vi "Grab with Software Trigger - LV2014.vi"() -> ()   [LabVIEW 2014]
doc: "The Grab VI acquires images continuously and displays the images in an image control using high-level acquisition VIs. A grab is appropriate for high-speed applications in which you need to process only one image at a time."
uses:
  <vilib>/vision/driver/NI_Vision_Acquisition_Software.lvlib
  <resource>/objmgr/imaqdx.rc
panel:
  in  "Timeout (ms)":u32=5000
  in  "Send Trigger":bool
  in  "Camera Name":refnum<k21> caption="IMAQdx Session"
  out "Buffer Number":u32
  out "Image":T1(plugin-control)
  out "Frame Rate":dbl(knob)=1.0526315789473684 scale=0.0..100.0
  in  "Stop":bool
  # "Overview: Demonstrates how to acquire images a Grab acquisition with software triggering.\nRequirements: Vision Acquisition Software\nInstructions: \n1. Select the Camera Name.\n2. Set Timeout (ms) to a value high enough to allow time to generate the trigger.\n3. Run the VI.\n4. Click Send Trigger to trigger the acquisition of a frame.\n5. After clicking Stop, VI will wait the timeout duration before stopping."
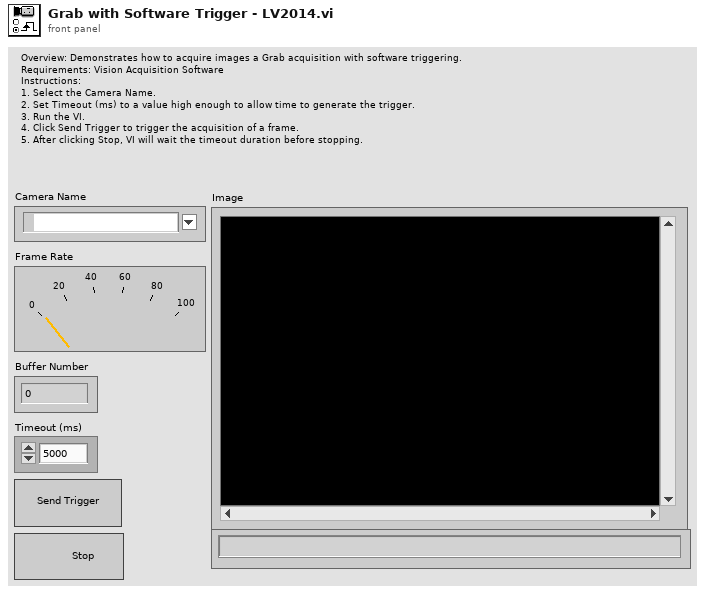
[diagram p1: front panel]
types:
  T1 = typedef "IMAQ Image.ctl" = refnum<image>
  T2 = typedef "IMAQdx.ctl" = refnum<k21>
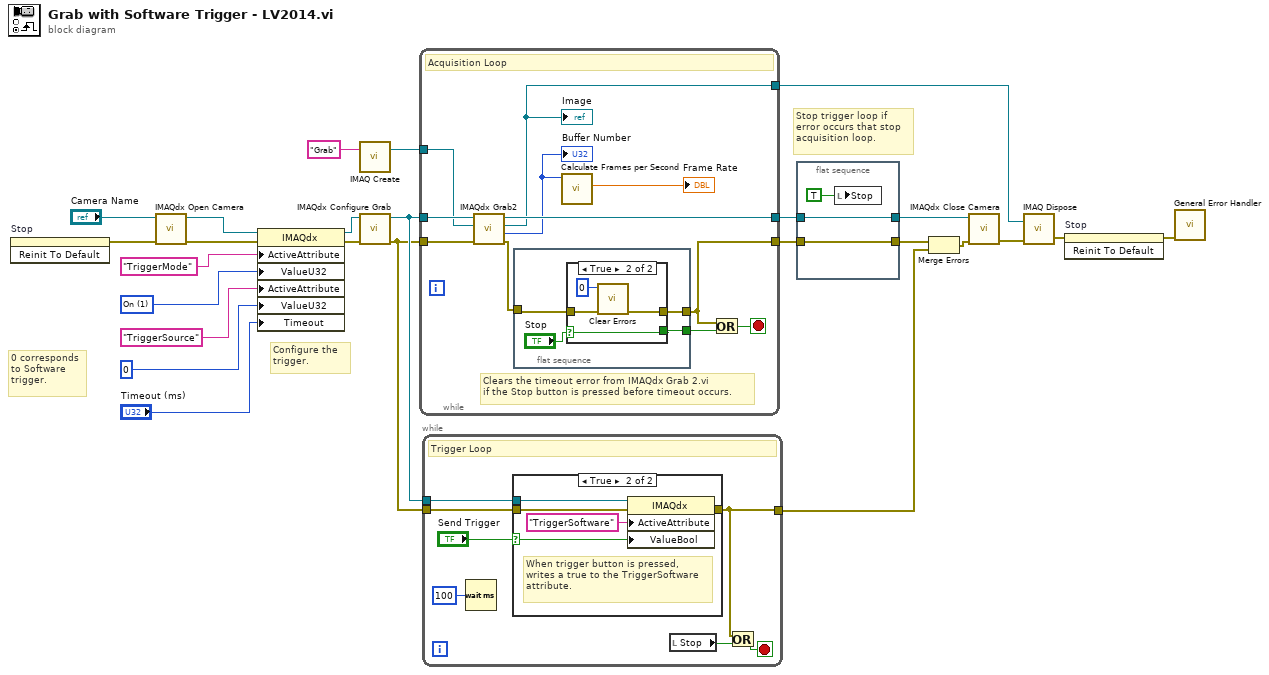
[diagram p0: block diagram]
diagram:
  w12 = u32 1 items=["Off", "On"] ("Trigger Mode")
  # "Configure the \ntrigger."
  # "Stop trigger loop if\nerror occurs that stop \nacquisition loop."
  # "0 corresponds\nto Software \ntrigger."
  n1 = invoke on="Stop" class="Bool (strict)" method="Reinit To Default"() -> (error out=w9:errorcluster)  [unwired: 3 in, 2 out]
  n2 = call <vilib>:"IMAQdx Open Camera.vi"("error in"=w9, "Session In"="Camera Name") -> ("error out"=w24:errorcluster, "Session Out"=w18:T2)  [unwired: 1 in, 7 out]
  n3 = property class="IMAQdx"(reference=w18, error in=w24, "ActiveAttribute"="TriggerMode", "ValueU32"=w12, "ActiveAttribute"="TriggerSource", "ValueU32"=u32 0, "Timeout"="Timeout (ms)") -> (reference out=w17:T2, error out=w19:errorcluster)
  n4 = call "IMAQ Create"("Image Name"="Grab") -> ("New Image"=w25:T1)  [unwired: 3 in, 2 out]
  n5 = call <vilib>:"IMAQdx Configure Grab.vi"("error in"=w19, "Session In"=w17) -> ("error out"=w10:errorcluster, "Session Out"=w11:T2)  [unwired: 8 out]
  n6 = while {
    tunnel: [w32] -> w8
    tunnel: w10 -> [w34]
    tunnel: w11 -> [w35]
    tunnel: [w26] -> w7
    tunnel: w25 -> [w33]
    tunnel: [w29] -> w22
    stop <- w36 stop-if-true
    # "Clears the timeout error from IMAQdx Grab 2.vi\nif the Stop button is pressed before timeout occurs."
    # "Acquisition Loop"
    n7 = call <vilib>:"IMAQdx Grab2.vi"("error in"=w34, "Image In"=w33, "Session In"=w35) -> ("error out"=w27:errorcluster, "Buffer Number Out"=w30:u32, "Image Out"=w29:T1, "Session Out"=w32:T2)  [unwired: 5 in]
    "Image" <- w29
    "Buffer Number" <- w30
    n8 = flat-sequence {
      tunnel: [w39] -> w28
      tunnel: w27 -> [w38]
      tunnel: [w37] -> w26
      frame #0 {
        n9 = case shown="True" "Stop" {
          selector: "Stop" -> [w41 w46]
          tunnel: [w41 w46] -> w39
          tunnel: w38 -> [w42 w45]
          tunnel: [w42 w44] -> w37
          frame False {
          }
          frame True {
            n10 = call <vilib>:"Clear Errors.vi"("error in (no error)"=w45, "specific error code to clear (0: all)"=0) -> ("error out"=w44:errorcluster)  [unwired: 4 in, 1 out]
          }
        }
      }
    }
    n11 = call <vilib>:"Calculate Frames per Second.vi"("Buffer Number"=w30) -> ("Processed Frames/s"=→"Frame Rate":dbl)  [unwired: 8 in, 2 out]
    n12 = Or(x=w26, y=w28) -> (x .or. y?=w36:bool)
  }
  n13 = while {
    tunnel: w11 -> [w52]
    tunnel: w10 -> [w51]
    tunnel: [w49] -> w1
    stop <- w50 stop-if-true
    # "Trigger Loop"
    n14 = Wait (ms)(milliseconds to wait=u32 100) -> ()  [unwired: 1 out]
    n15 = case shown="True" "Send Trigger" {
      selector: "Send Trigger" -> [_ w55]
      tunnel: w52 -> [_ w59]
      tunnel: w51 -> [w54 w58]
      tunnel: [w54 w57] -> w49
      frame False {
      }
      frame True {
        # "When trigger button is pressed,\nwrites a true to the TriggerSoftware\nattribute."
        n16 = property class="IMAQdx"(reference=w59, error in=w58, "ActiveAttribute"="TriggerSoftware", "ValueBool"=w55) -> (error out=w57:errorcluster)  [unwired: 1 out]
      }
    }
    n17 = local read "Stop"() -> (w53:bool)
    n18 = Or(x=w49, y=w53) -> (x .or. y?=w50:bool)
  }
  n19 = flat-sequence {
    tunnel: w8 -> [w60]
    tunnel: w7 -> [w61]
    tunnel: [w61] -> w6
    tunnel: [w60] -> w5
    frame #0 {
      n20 = local write "Stop"(TRUE ("Stop")) -> ()
    }
  }
  n21 = Merge Errors(w6, w1) -> (w2:errorcluster)
  n22 = call <vilib>:"IMAQdx Close Camera.vi"("error in"=w2, "Session In"=w5) -> ("error out"=w21:errorcluster)  [unwired: 9 out]
  n23 = call "IMAQ Dispose"("Image"=w22, "error in (no error)"=w21) -> ("error out"=w4:errorcluster)  [unwired: 4 in]
  n24 = invoke on="Stop" class="Bool (strict)" method="Reinit To Default"(error in=w4) -> (error out=w3:errorcluster)  [unwired: 2 in, 2 out]
  n25 = call <vilib>:"General Error Handler.vi"("error in (no error)"=w3) -> ()  [unwired: 2 in, 13 out]
